vi "CRYCalc Weighting.vi"(9 "Weight":cluster{"x":dbl, "y":dbl}[](array[cluster]), 10 "df":dbl format="%.2f", 11 "Complex FFT (Vrms)":cdb[](array[numeric]) format="%.2f") -> (3 "Weighted Com":cdb[](array[numeric]))   [LabVIEW 2013]
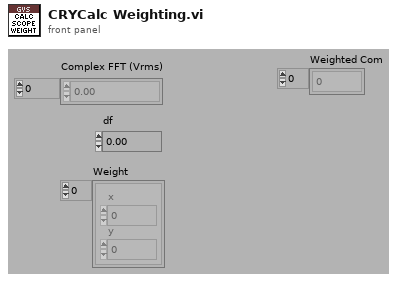
[diagram p1: front panel]
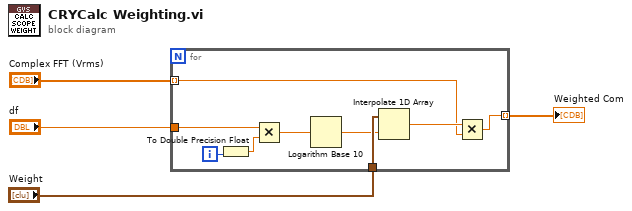
[diagram p0: block diagram]
diagram:
  n1 = for {
    tunnel: "Complex FFT (Vrms)" -> [w9] mode=indexing
    tunnel: "df" -> [w13]
    tunnel: "Weight" -> [w10]
    tunnel: [w8] -> w2 mode=indexing
    i -> [w12]
    n2 = To Double Precision Float(number=w12) -> (double precision float=w7:dbl)
    n3 = Multiply(x=w13, y=w7) -> (x*y=w6:dbl)
    n4 = Logarithm Base 10(1:w6) -> (0:w5:dbl)
    n5 = Interpolate 1D Array(1:w5, 2:w10) -> (0:w11:dbl)
    n6 = Multiply(x=w11, y=w9) -> (x*y=w8:cdb)
  }
  "Weighted Com" <- w2
